vi "Find Average Center.vi"(7 "Tray Number":i32, 9 "XYZTheta":dbl[](array[numeric]), 11 "Gantry In":refnum<k24>) -> (1 "XYZTheta Centers":dbl[][](array[numeric]), 3 "Gantry Out":refnum<k24>)   [LabVIEW 2019, in "Assembly Tray.lvclass"]
uses:
  Assembly Tray.lvclass
  Controller/Camera/Machine Vision.ctl
  C:/Program Files (x86)/Aerotech/A3200/LabVIEW/2010/Bin/Aerotech.A3200.dll
  Program Files (x86)/Aerotech/A3200/LabVIEW/2010/Bin/Aerotech.A3200.dll
  Find Tray.ctl
  Controller/Camera/Camera settings.ctl
  Controller/Camera/Image processing.ctl
  Controller/Camera/Camera.lvclass
  Controller/Motion/A3200/A3200.lvclass
panel:
  in  "Image processing":T1={"Brightness"=128.0, "Contrast"=45.0, "Gamma"=1.0471123} {"Brightness" scale=0.0..400.0; "Contrast" scale=0.0..90.0; "Gamma" scale=0.005..5.0}
  in  "Camera settings":T2={"Gamma"=1.6, "Gain"=0, "Sharpness"=0, "Contrast"=0.0, "Exposure"=0.0078125} {"Exposure" min=0.000244140625 max=0.5 scale=0.0002..0.5; "Contrast" min=0.0 max=1.0 scale=0.001..1.0; "Sharpness" min=0 max=2 step=1 scale=0.0..2.0; "Gain" min=0 max=100 step=1 scale=0.1..100.0; "Gamma" min=0.01 max=10.0 scale=0.01..10.0}
  in  "Override presets":bool
  out "Center":dbl[](array[numeric])
  out "Syringe Area":dbl[](array[numeric])
  in  "Go to Syringe Area":bool
  in  "Record Syringe Area":bool
  in  "Carrier Tray":T3
  in  "Position":bool=TRUE
  in  "Go to Center":bool
  in  "Joystick":bool
  in  "Record Bottom Left":bool
  in  "Record Top Right":bool
  in  "Record Top Left":bool
  in  "Record Bottom Right":bool
  out "TR XY":dbl[](array[numeric])
  out "BR XY":dbl[](array[numeric])
  out "BL XY":dbl[](array[numeric])
  out "TL XY":dbl[](array[numeric])
  in  "Go to Top Left":bool
  in  "Go to Bottom Left":bool
  in  "Go to Top Right":bool
  in  "Go to Bottom Right":bool
  out "Gantry":dbl[](array[numeric])
  out "Sum":dbl[](array[numeric])
  in  "Stop Program":bool
  out "Image":T4(plugin-control)
  out "Camera":dbl[](array[numeric])
  in  "Machine Vision":T5
  # "1"
  # "2"
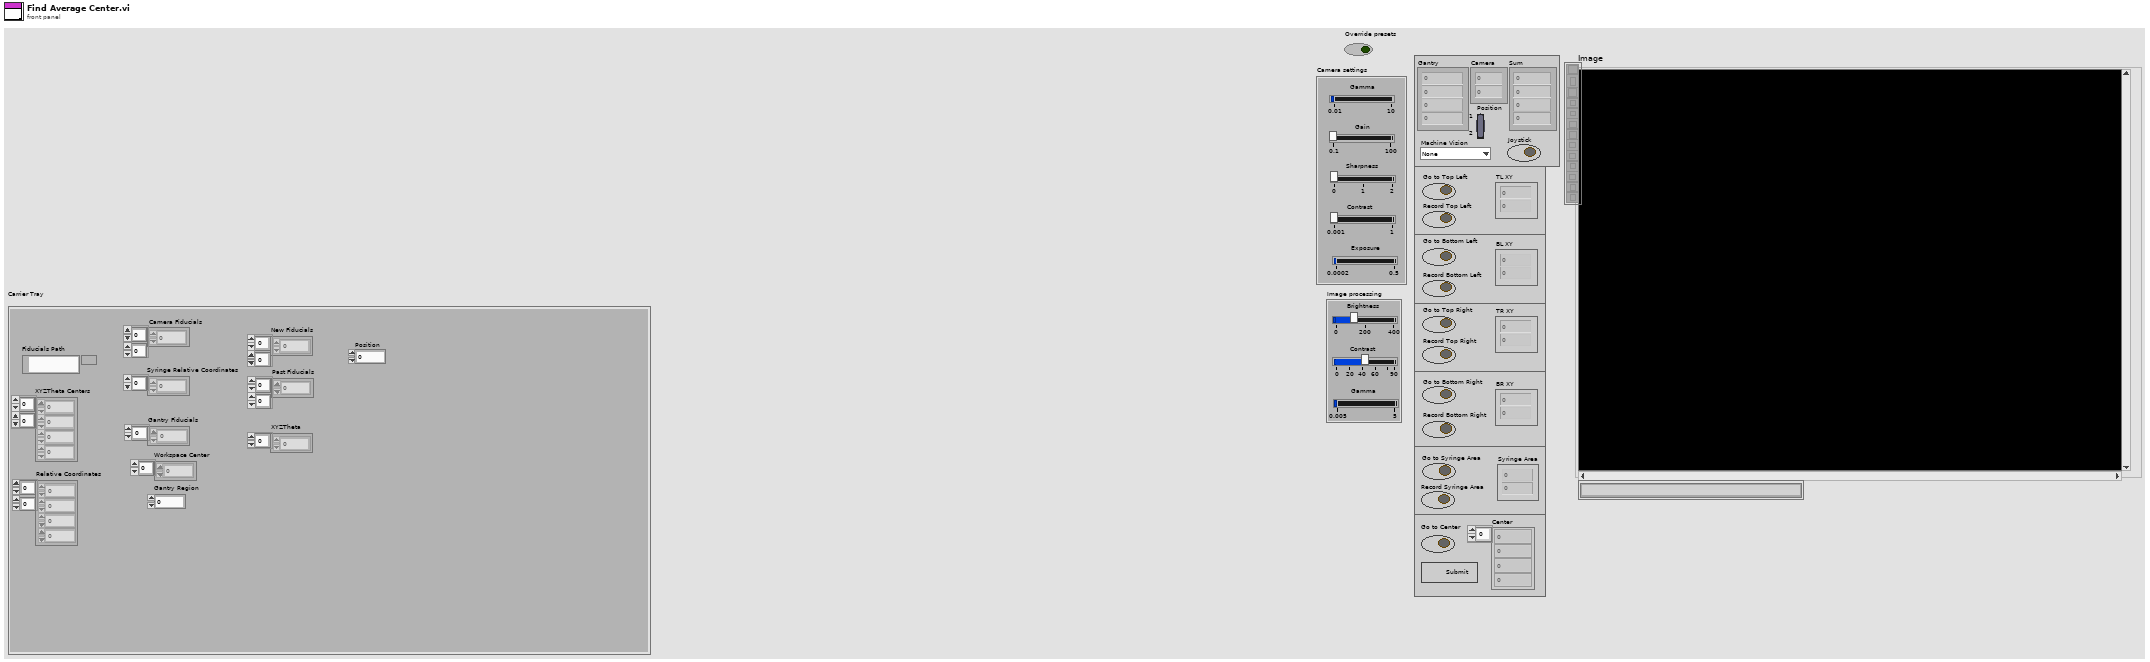
[diagram p1: front panel]
types:
  T1 = typedef "Camera.lvclass/Image processing.ctl" = cluster{"Brightness":sgl, "Contrast":sgl, "Gamma":sgl}
  T2 = typedef "Camera.lvclass/Camera settings.ctl" = cluster{"Gamma":dbl, "Gain":i64, "Sharpness":i64, "Contrast":dbl, "Exposure":dbl}
  T3 = typedef "Assembly Tray.lvclass/Find Tray.ctl" = cluster{"Gantry Fiducials":dbl[], "Relative Coordinates":dbl[][], "Camera Fiducials":dbl[][], "XYZTheta Centers":dbl[][], "Workspace Center":dbl[], "Syringe Relative Coordinates":dbl[], "Gantry Region":dbl, "Fiducials Path":path, "New Fiducials":dbl[][], "Past Fiducials":dbl[][], "XYZTheta":dbl[], "Position":i32}
  T4 = typedef "IMAQ Image.ctl" = refnum<image>
  T5 = typedef "Camera.lvclass/Machine Vision.ctl" = enum16{"None", "Tray Fiducials", "HPK Silicon", "Hexaboard", "Corner (TL, BR)", "Corner (BL, TR)", "sensor TL", "sensor BL", "sensor TR", "sensor BR", "hexaboard TL", "hexaboard BL", "hexaboard TR", "hexaboard BR"}
  T6 = typedef "File Paths.ctl" = cluster{"Glue Pattern Folder":path, "Carrier Tray Folder":path, "Pick Up Tool Fixture Folder":path, "Components Folder":path, "Bellows Tool Offset.txt":path, "Pick Up Tool Offset.txt":path, "Dispense Tip Offset.txt":path, "Log Files":path}
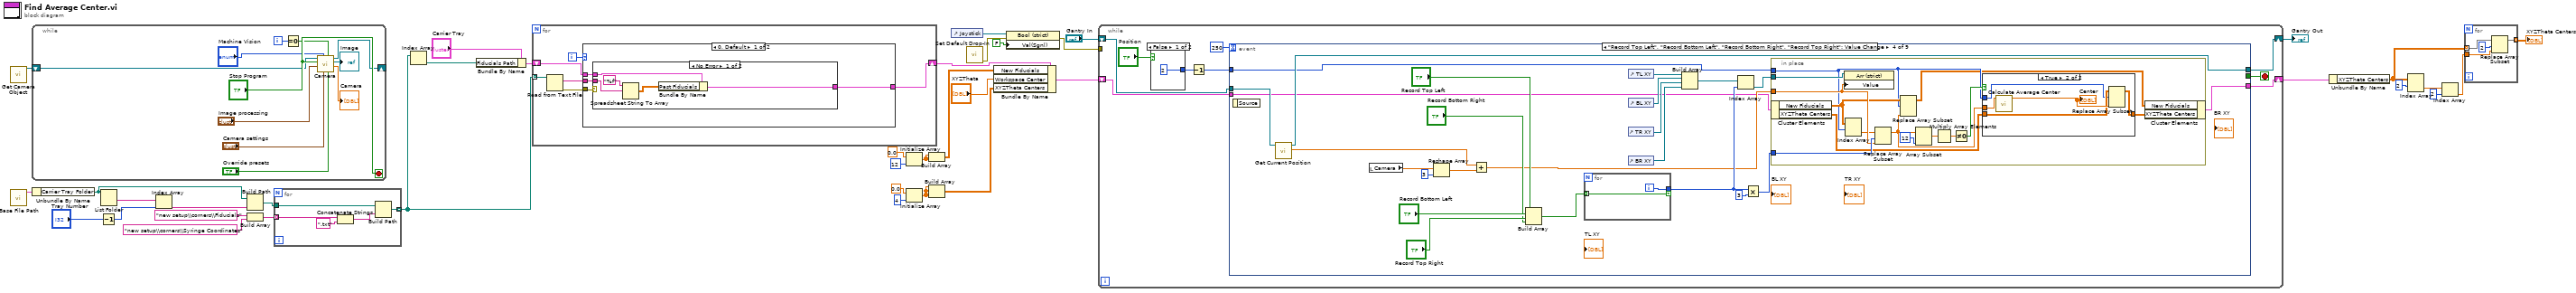
[diagram p0: block diagram]
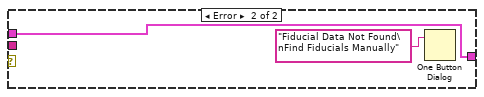
[diagram p2: hidden frame]
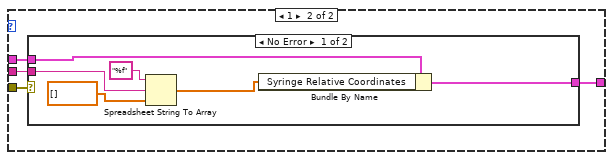
[diagram p3: hidden frame]
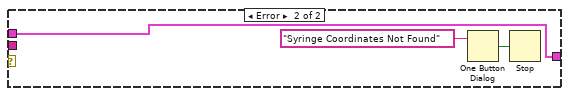
[diagram p4: hidden frame]
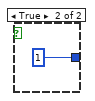
[diagram p5: hidden frame]
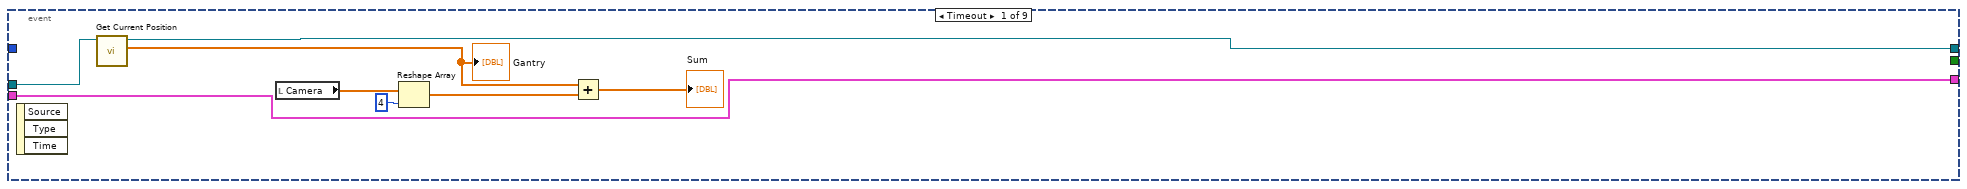
[diagram p6: hidden frame]
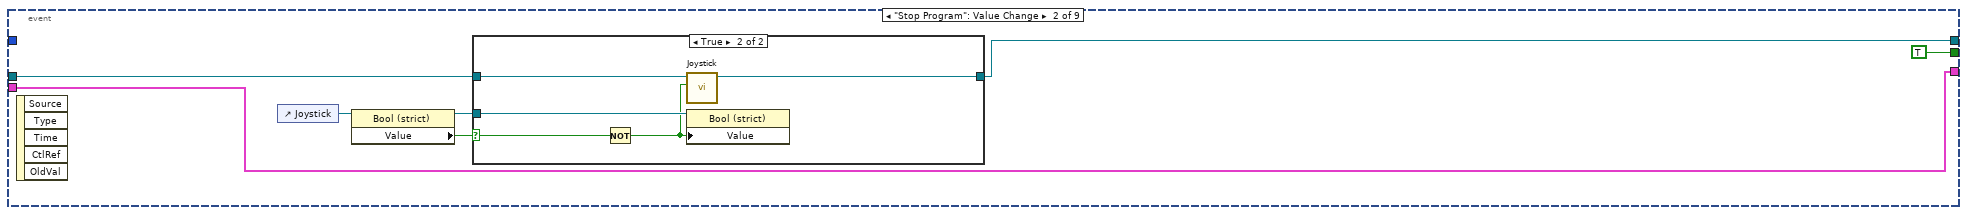
[diagram p7: hidden frame]
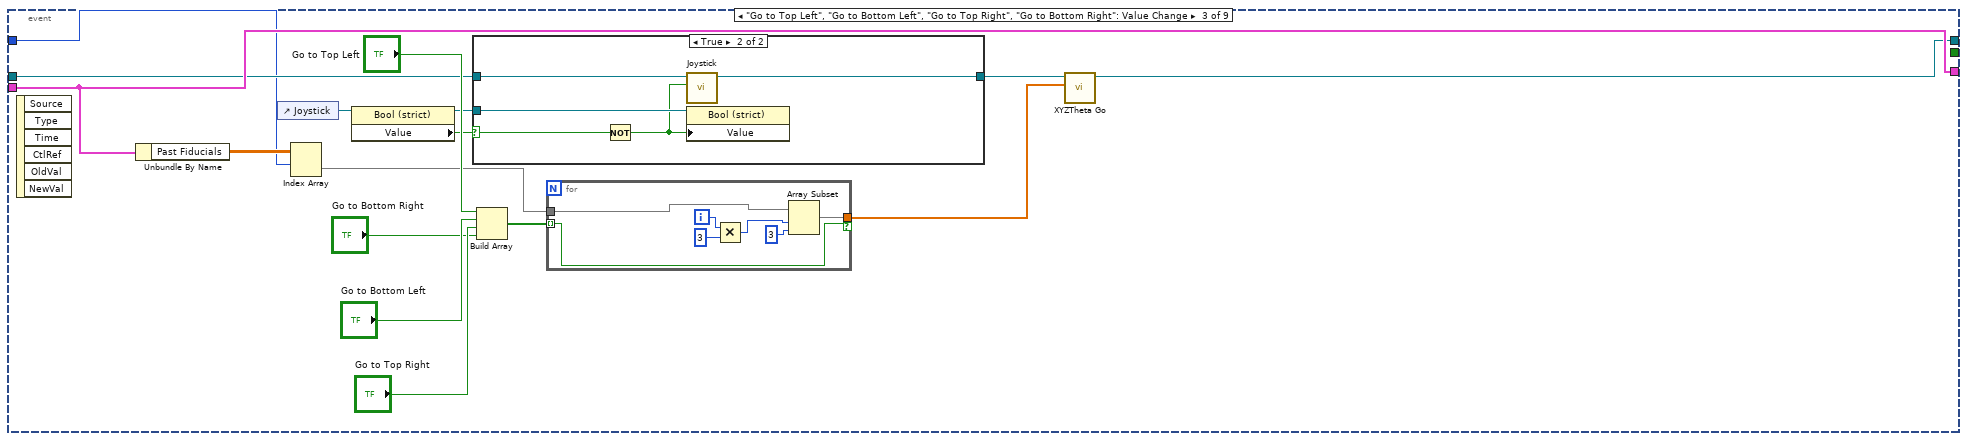
[diagram p9: hidden frame]
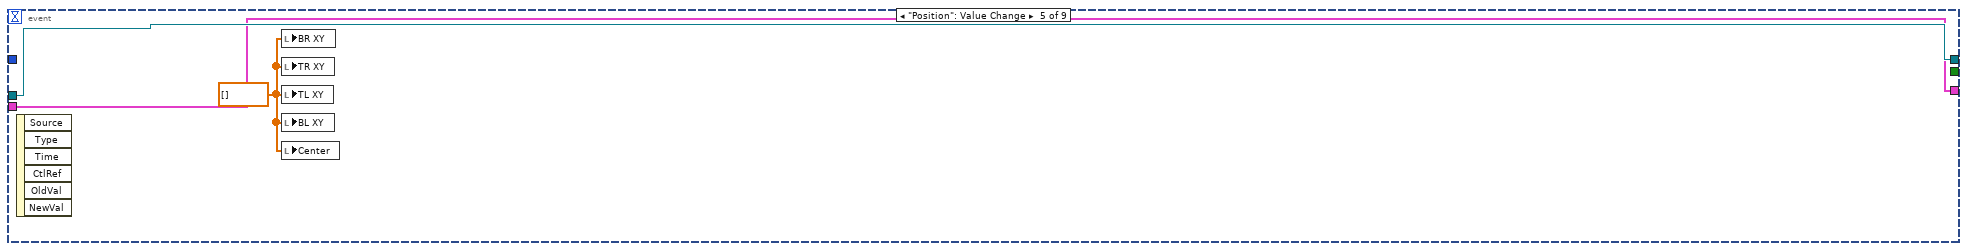
[diagram p12: hidden frame]
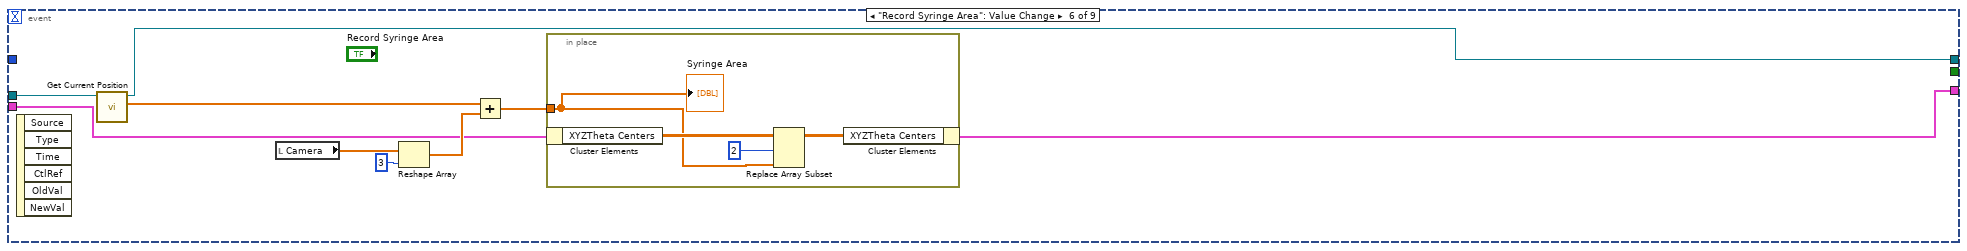
[diagram p13: hidden frame]
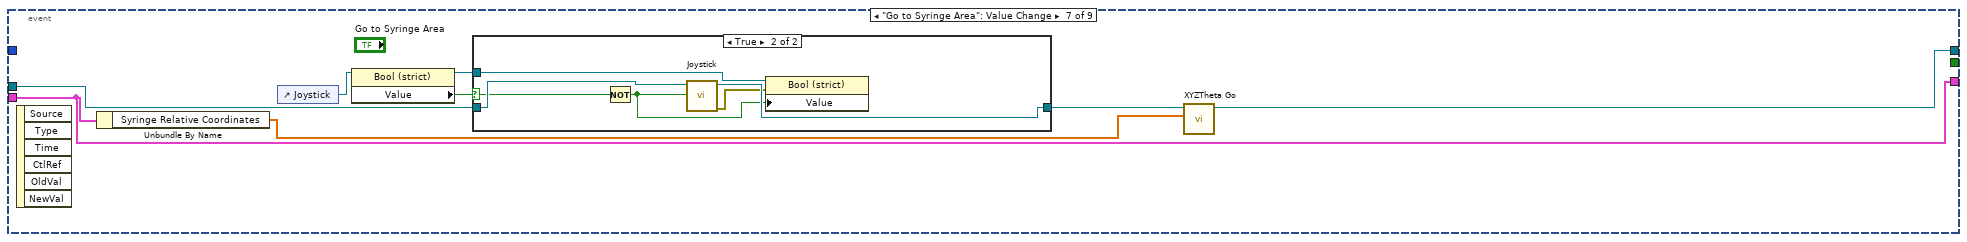
[diagram p14: hidden frame]
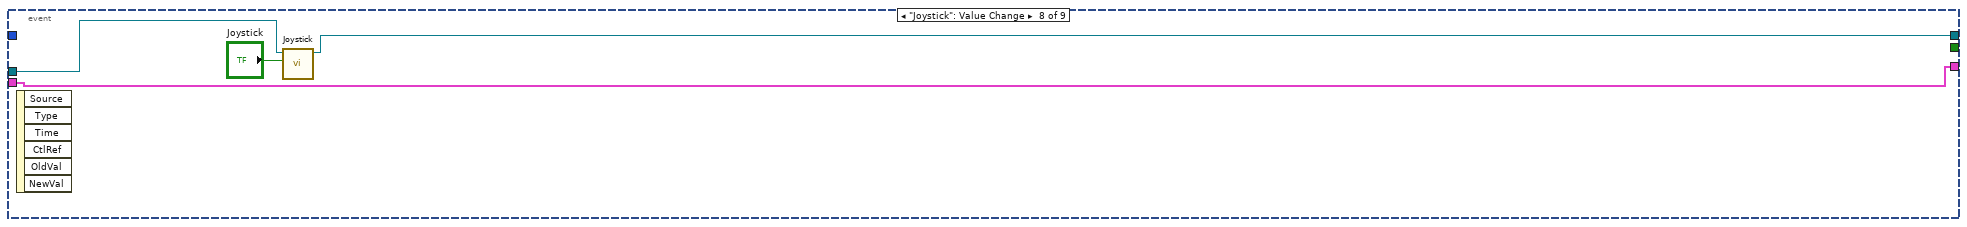
[diagram p16: hidden frame]
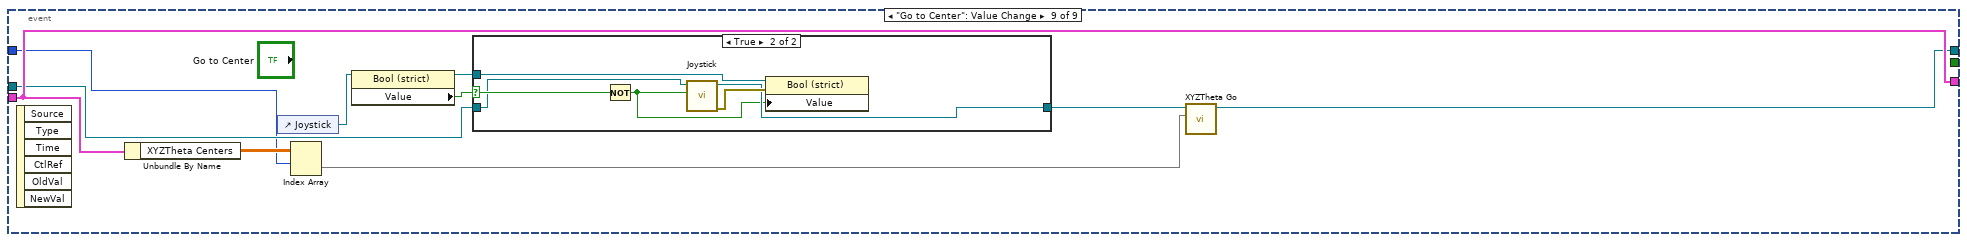
[diagram p17: hidden frame]
diagram:
  n1 = call "Get Camera Object.vi"() -> ("Camera out"=w1:refnum<class "Camera.lvclass">)  [unwired: 10 in, 1 out]
  n2 = call "Base File Path.vi"() -> ("Paths Out"=w22:T6)  [unwired: 11 in]
  n3 = while {
    shift-right: [w45] -> _
    shift-left: w1 -> [w49]
    i -> [w41]
    stop <- "Stop Program" stop-if-true
    n4 = Equal To 0?(x=w41) -> (x = 0?=w40:bool)
    n5 = call "Camera.vi"("Override presets"="Override presets", "Loop 0"=w40, "Camera settings"="Camera settings", "Machine Vision"="Machine Vision", "BCG Image Processing"="Image processing", "Stop"="Stop Program", "Camera in"=w49) -> ("Camera"=→"Camera":dbl[], "Image"=→"Image":T4, "Camera out"=w45:refnum<class "Camera.lvclass">)  [unwired: 1 in, 1 out]
  }
  n6 = Unbundle By Name(w22) -> ("Carrier Tray Folder"=w20:path)
  n7 = Decrement(x="Tray Number") -> (x-1=w21:i32)
  n8 = List Folder(path=w20) -> (folder names=w24:string[])  [unwired: 3 in, 3 out]
  n9 = Index Array(array=w24, index=w21) -> (element=w23:string)
  n10 = Build Path(base path=w20, name or relative path=w23) -> (appended path=w26:path)
  n11 = Build Array("new setup\\corners\\Fiducials" ("format string"), "new setup\\corners\\Syringe Coordinates" ("element")) -> (w25:string[])
  n12 = for {
    tunnel: w25 -> [w53] mode=indexing
    tunnel: w26 -> [w55]
    tunnel: [w54] -> w19 mode=indexing
    n13 = Concatenate Strings(w53, ".txt" ("string")) -> (w51:string)
    n14 = Build Path(base path=w55, name or relative path=w51) -> (appended path=w54:path)
  }
  n15 = Index Array(array=w19) -> (element=w27:path)  [unwired: 1 in]
  n16 = Bundle By Name(cluster="Carrier Tray", "Fiducials Path"=w27) -> (w29:T3)
  n17 = for {
    tunnel: w19 -> [w60] mode=indexing
    shift-right: [w56] -> w16
    shift-left: w29 -> [w57]
    i -> [w58]
    n18 = Read from Text File(file (use dialog)=w60) -> (text=w61:string, error out=w59:errorcluster)  [unwired: 3 in, 2 out]
    n19 = case shown="0, Default" w58 {
      tunnel: w61 -> [w65 w74]
      tunnel: w59 -> [w64 w75]
      tunnel: w57 -> [w63 w76]
      tunnel: [w62 w73] -> w56
      frame 0, Default {
        n20 = case shown="No Error" w64 {
          tunnel: w65 -> [w69 _]
          tunnel: w63 -> [w67 w71]
          tunnel: [w68 w71] -> w62
          frame No Error {
            n21 = Spreadsheet String To Array(format string="%f", spreadsheet string=w69) -> (array=w66:dbl[][])  [unwired: 2 in]
            n22 = Bundle By Name(cluster=w67, "Past Fiducials"=w66) -> (w68:T3)
          }
          frame Error {
            n23 = One Button Dialog(message="Fiducial Data Not Found\nFind Fiducials Manually") -> ()  [unwired: 1 in, 1 out]
          }
        }
      }
      frame 1 {
        n24 = case shown="No Error" w75 {
          tunnel: w74 -> [w80 _]
          tunnel: [w78 w83] -> w73
          tunnel: w76 -> [w79 w83]
          frame No Error {
            n25 = Spreadsheet String To Array(format string="%f", spreadsheet string=w80, array type (2D Dbl)=dbl[] []) -> (array=w77:dbl[])  [unwired: 1 in]
            n26 = Bundle By Name(cluster=w79, "Syringe Relative Coordinates"=w77) -> (w78:T3)
          }
          frame Error {
            n27 = One Button Dialog(message="Syringe Coordinates Not Found") -> (true=w84:bool)  [unwired: 1 in]
            n28 = Stop(stop? (T)=w84) -> ()
          }
        }
      }
    }
  }
  n29 = Initialize Array(0.0 ("element"), 12 ("dimension size")) -> (w13:dbl[])
  n30 = Initialize Array(0.0 ("element"), 4 ("dimension size")) -> (w9:dbl[])
  n31 = Build Array(w13, w13) -> (w14:dbl[][])
  n32 = Build Array(w9, w9, w9) -> (w8:dbl[][])
  n33 = control-ref of="Joystick"() -> (w38:refnum<vi>)
  n34 = call "Set Default Drop-In.vi"() -> ("error out"=w32:errorcluster)  [unwired: 11 in]
  n35 = Bundle By Name(cluster=w16, "New Fiducials"=w14, "Workspace Center"="XYZTheta", "XYZTheta Centers"=w8) -> (w39:T3)
  n36 = property class="Bool (strict)"(reference=w38, error in=w32, "Val(Sgnl)"=FALSE) -> (error out=w36:errorcluster)  [unwired: 1 out]
  n37 = while {
    shift-right: [w86] -> w12
    shift-left: w39 -> [w93]
    tunnel: w36 -> [_]
    shift-right: [w90] -> w30
    shift-left: "Gantry In" -> [w91]
    stop <- w94 stop-if-true
    n38 = case shown="False" "Position" {
      tunnel: [2 1] -> w87
      frame False {
      }
      frame True {
      }
    }
    n39 = Decrement(x=w87) -> (x-1=w89:i32)
    n40 = event shown="[3] \"Record Top Left\", \"Record Bottom Left\", \"Record Bottom Right\", \"Record Top Right\": Value Change" {
      selector: _ -> [_ _ _ _ _ _ _ _ _]
      dyn-events: _ -> [_ _ _ _ _ _ _ _ _]
      timeout: 250 -> [_ _ _ _ _ _ _ _ _]
      tunnel: [_ TRUE _ _ _ _ _ _ _] -> w94
      tunnel: w93 -> [w103 w106 w127 w148 w194 w198 w216 w227 w237]
      tunnel: [w103 w106 w127 w170 w194 w197 w216 w227 w237] -> w86
      tunnel: w91 -> [w99 w107 w124 w151 w195 w204 w213 w226 w233]
      tunnel: [w98 w105 w121 w149 w195 w199 w215 w224 w231] -> w90
      tunnel: w89 -> [_ _ w118 w147 _ _ _ _ w229]
      event Timeout {
        n41 = event-data() -> ()  [unwired: 1 in, 3 out]
        n42 = call "Get Current Position.vi"("Gantry In"=w99) -> ("XYZTheta Out"=w97:dbl[], "Gantry Out"=w98:refnum<k24>)  [unwired: 8 in, 1 out]
        "Gantry" <- w97
        n43 = local read "Camera"() -> (w102:dbl[])
        n44 = Reshape Array(w102, 4 ("dimension size")) -> (w100:dbl[])
        n45 = Add(x=w97, y=w100) -> (x+y=→"Sum":dbl[])
      }
      event "Stop Program": Value Change {
        n46 = event-data() -> ()  [unwired: 1 in, 5 out]
        n47 = control-ref of="Joystick"() -> (w108:refnum<vi>)
        n48 = property class="Bool (strict)"(reference=w108) -> (reference out=w109:refnum<vi>, "Value"=w110:bool)  [unwired: 1 in, 1 out]
        n49 = case shown="True" w110 {
          selector: w110 -> [_ w117]
          tunnel: w107 -> [w112 w115]
          tunnel: [w112 w114] -> w105
          tunnel: w109 -> [_ w116]
          frame False {
          }
          frame True {
            n50 = Not(x=w117) -> (.not. x?=w113:bool)
            n51 = call "Joystick.vi"("Joystick"=w113, "Gantry In"=w115) -> ("Gantry Out"=w114:refnum<k24>)  [unwired: 8 in, 1 out]
            n52 = property class="Bool (strict)"(reference=w116, "Value"=w113) -> ()  [unwired: 1 in, 2 out]
          }
        }
      }
      event "Go to Top Left", "Go to Bottom Left", "Go to Top Right", "Go to Bottom Right": Value Change {
        n53 = event-data() -> ()  [unwired: 1 in, 6 out]
        n54 = Unbundle By Name(w127) -> ("Past Fiducials"=w120:dbl[][])
        n55 = control-ref of="Joystick"() -> (w122:refnum<vi>)
        n56 = Index Array(array=w120, index (row)=w118) -> (element=w119:dbl[])  [unwired: 1 in]
        n57 = property class="Bool (strict)"(reference=w122) -> (reference out=w125:refnum<vi>, "Value"=w126:bool)  [unwired: 1 in, 1 out]
        n58 = case shown="True" w126 {
          selector: w126 -> [_ w139]
          tunnel: w124 -> [w134 w137]
          tunnel: [w134 w135] -> w123
          tunnel: w125 -> [_ w138]
          frame False {
          }
          frame True {
            n59 = Not(x=w139) -> (.not. x?=w136:bool)
            n60 = call "Joystick.vi"("Joystick"=w136, "Gantry In"=w137) -> ("Gantry Out"=w135:refnum<k24>)  [unwired: 8 in, 1 out]
            n61 = property class="Bool (strict)"(reference=w138, "Value"=w136) -> ()  [unwired: 1 in, 2 out]
          }
        }
        n62 = Build Array("Go to Top Left", "Go to Bottom Left", "Go to Top Right", "Go to Bottom Right") -> (w129:bool[])
        n63 = for {
          tunnel: w129 -> [w146] mode=indexing
          tunnel: w119 -> [w145]
          tunnel: [w140] -> w128 if=w146
          i -> [w143]
          n64 = Multiply(x=w143, y=3) -> (x*y=w141:i32)
          n65 = Array Subset(array=w145, index=w141, length=3) -> (w140:dbl[])
        }
        n66 = call "XYZTheta Go.vi"("XYZTheta In"=w128, "Gantry In"=w123) -> ("Gantry Out"=w121:refnum<k24>)  [unwired: 7 in, 2 out]
      }
      event "Record Top Left", "Record Bottom Left", "Record Bottom Right", "Record Top Right": Value Change {
        n67 = event-data() -> ()  [unwired: 1 in, 1 out]
        n68 = call "Get Current Position.vi"("Gantry In"=w151) -> ("XYZTheta Out"=w150:dbl[], "Gantry Out"=w149:refnum<k24>)  [unwired: 8 in, 1 out]
        n69 = local read "Camera"() -> (w154:dbl[])
        n70 = Reshape Array(w154, 3 ("dimension size")) -> (w153:dbl[])
        n71 = Add(x=w150, y=w153) -> (x+y=w152:dbl[])
        n72 = Build Array("Record Top Left", "Record Bottom Left", "Record Top Right", "Record Bottom Right") -> (w165:bool[])
        n73 = for {
          tunnel: w165 -> [w171] mode=indexing
          tunnel: [w172] -> w157 if=w171
          i -> [w172]
        }
        n74 = control-ref of="TL XY"() -> (w164:refnum<vi>)
        n75 = control-ref of="BL XY"() -> (w163:refnum<vi>)
        n76 = control-ref of="TR XY"() -> (w162:refnum<vi>)
        n77 = control-ref of="BR XY"() -> (w161:refnum<vi>)
        n78 = Build Array(w164, w163, w162, w161) -> (w160:refnum<vi>[])
        n79 = Index Array(array=w160, index=w157) -> (element=w159:refnum<vi>)
        n80 = Multiply(x=w157, y=3) -> (x*y=w155:i32)
        n81 = in-place {
          in-place-border: w155 -> [w186]
          in-place-border: w159 -> [w184]
          in-place-border: w152 -> [w183]
          in-place-border: w147 -> [w174]
          n82 = in-place-cluster #1(w148) -> ("New Fiducials"=w175:dbl[][], "XYZTheta Centers"=w177:dbl[][])
          n83 = property class="Arr (strict)"(reference=w184, "Value"=w183) -> ()  [unwired: 1 in, 2 out]
          n84 = Index Array(array=w175, index (row)=w174) -> (element=w178:dbl[])  [unwired: 1 in]
          n85 = Replace Array Subset(array=w178, new element=w183, index=w186) -> (w182:dbl[])
          n86 = Replace Array Subset(array=w175, new element=w182, index (row)=w174) -> (w173:dbl[][])  [unwired: 1 in]
          n87 = Array Subset(array=w182, length=12) -> (w180:dbl[])  [unwired: 1 in]
          n88 = Multiply Array Elements(1:w180) -> (0:w179:dbl)
          n89 = Not Equal To 0?(x=w179) -> (x != 0?=w185:bool)
          n90 = case shown="True" w185 {
            tunnel: w182 -> [_ w189]
            tunnel: w177 -> [w187 w191]
            tunnel: w174 -> [_ w188]
            tunnel: [w187 w190] -> w176
            frame False {
            }
            frame True {
              n91 = call "Calculate Average Center.vi"("Gantry Fiducials"=w189) -> ("XYZTheta"=w192:dbl[])  [unwired: 10 in]
              "Center" <- w192
              n92 = Replace Array Subset(array=w191, new element=w192, index (row)=w188) -> (w190:dbl[][])  [unwired: 1 in]
            }
          }
          n93 = in-place-cluster #1("New Fiducials"=w173, "XYZTheta Centers"=w176) -> (w170:T3)
        }
      }
      event "Position": Value Change {
        w193 = dbl[] [] ("TR XY")
        n94 = event-data() -> ()  [unwired: 1 in, 6 out]
        n95 = local write "BR XY"(w193) -> ()
        n96 = local write "TR XY"(w193) -> ()
        n97 = local write "TL XY"(w193) -> ()
        n98 = local write "BL XY"(w193) -> ()
        n99 = local write "Center"(w193) -> ()
      }
      event "Record Syringe Area": Value Change {
        n100 = event-data() -> ()  [unwired: 1 in, 6 out]
        n101 = call "Get Current Position.vi"("Gantry In"=w204) -> ("XYZTheta Out"=w200:dbl[], "Gantry Out"=w199:refnum<k24>)  [unwired: 8 in, 1 out]
        n102 = local read "Camera"() -> (w201:dbl[])
        n103 = Reshape Array(w201, 3 ("dimension size")) -> (w202:dbl[])
        n104 = Add(x=w200, y=w202) -> (x+y=w196:dbl[])
        n105 = in-place {
          in-place-border: w196 -> [w207]
          n106 = in-place-cluster #2(w198) -> ("XYZTheta Centers"=w208:dbl[][])
          n107 = Replace Array Subset(array=w208, new element=w207, index (row)=2) -> (w205:dbl[][])  [unwired: 1 in]
          n108 = in-place-cluster #2("XYZTheta Centers"=w205) -> (w197:T3)
          "Syringe Area" <- w207
        }
      }
      event "Go to Syringe Area": Value Change {
        n109 = event-data() -> ()  [unwired: 1 in, 6 out]
        n110 = Unbundle By Name(w216) -> ("Syringe Relative Coordinates"=w209:dbl[])
        n111 = control-ref of="Joystick"() -> (w212:refnum<vi>)
        n112 = property class="Bool (strict)"(reference=w212) -> (reference out=w210:refnum<vi>, "Value"=w211:bool)  [unwired: 1 in, 1 out]
        n113 = case shown="True" w211 {
          selector: w211 -> [_ w219]
          tunnel: [w217 w223] -> w214
          tunnel: w213 -> [w217 w222]
          tunnel: w210 -> [_ w221]
          frame False {
          }
          frame True {
            n114 = Not(x=w219) -> (.not. x?=w218:bool)
            n115 = call "Joystick.vi"("Joystick"=w218, "Gantry In"=w222) -> ("error out"=w220:errorcluster, "Gantry Out"=w223:refnum<k24>)  [unwired: 8 in]
            n116 = property class="Bool (strict)"(reference=w221, error in=w220, "Value"=w218) -> ()  [unwired: 2 out]
          }
        }
        n117 = call "XYZTheta Go.vi"("XYZTheta In"=w209, "Gantry In"=w214) -> ("Gantry Out"=w215:refnum<k24>)  [unwired: 7 in, 2 out]
      }
      event "Joystick": Value Change {
        n118 = event-data() -> ()  [unwired: 1 in, 6 out]
        n119 = call "Joystick.vi"("Joystick"="Joystick", "Gantry In"=w226) -> ("Gantry Out"=w224:refnum<k24>)  [unwired: 8 in, 1 out]
      }
      event "Go to Center": Value Change {
        n120 = event-data() -> ()  [unwired: 1 in, 6 out]
        n121 = Unbundle By Name(w237) -> ("XYZTheta Centers"=w230:dbl[][])
        n122 = control-ref of="Joystick"() -> (w234:refnum<vi>)
        n123 = Index Array(array=w230, index (row)=w229) -> (element=w228:dbl[])  [unwired: 1 in]
        n124 = property class="Bool (strict)"(reference=w234) -> (reference out=w235:refnum<vi>, "Value"=w236:bool)  [unwired: 1 in, 1 out]
        n125 = case shown="True" w236 {
          selector: w236 -> [_ w244]
          tunnel: w233 -> [w238 w241]
          tunnel: [w238 w240] -> w232
          tunnel: w235 -> [_ w243]
          frame False {
          }
          frame True {
            n126 = Not(x=w244) -> (.not. x?=w239:bool)
            n127 = call "Joystick.vi"("Joystick"=w239, "Gantry In"=w241) -> ("error out"=w242:errorcluster, "Gantry Out"=w240:refnum<k24>)  [unwired: 8 in]
            n128 = property class="Bool (strict)"(reference=w243, error in=w242, "Value"=w239) -> ()  [unwired: 2 out]
          }
        }
        n129 = call "XYZTheta Go.vi"("XYZTheta In"=w228, "Gantry In"=w232) -> ("Gantry Out"=w231:refnum<k24>)  [unwired: 7 in, 2 out]
      }
    }
  }
  "Gantry Out" <- w30
  n130 = Unbundle By Name(w12) -> ("XYZTheta Centers"=w4:dbl[][])
  n131 = Index Array(array=w4, index (row)=2) -> (element=w6:dbl[])  [unwired: 1 in]
  n132 = Index Array(array=w6, index=2) -> (element=w3:dbl)
  n133 = for {
    tunnel: w4 -> [w248] mode=indexing
    tunnel: w3 -> [w247]
    tunnel: [w246] -> w2 mode=indexing
    n134 = Replace Array Subset(array=w248, new element=w247, index=2) -> (w246:dbl[])
  }
  "XYZTheta Centers" <- w2
